vi "Add Sink.vi"(4 "Sink Name":string, 6 "Log Sink Reference":refnum<data-value>, 8 "error in (no error)":errorcluster, 11 "Application Log in":refnum<class "Application Log.lvclass">) -> (0 "error out":errorcluster, 3 "Application Log out":refnum<class "Application Log.lvclass">)   [LabVIEW 2016, in "Stream Log.lvlib" / "Application Log.lvclass"]
doc: "--\nCopyright © 2017 Composed SystemsI All rights reserved.\n\nAuthor: Jon McBee <jon.mcbee@composed.io>\n\nThis library is provided \"AS IS\" ,WITHOUT WARRANTIES OR\nCONDITIONS OF ANY KIND, either express or implied.\n\nComposed Systems -- composed.io\n\nStream 0.0.1.1\nJon McBee - Composed Systems\nCopyright (c) 2017, Composed Systems"
uses:
  <userlib>/Composed Systems/Stream/Log/Application Log/Application Log.lvclass
  <userlib>/Composed Systems/Stream/Log/Log Sink/Log Sink.lvclass
  <userlib>/Composed Systems/Stream/Log/Application Log/Application Log.lvclass/Application Log.ctl
  <userlib>/Composed Systems/Stream/Log/Sink Look Up Table/Sink Look Up Table.lvclass
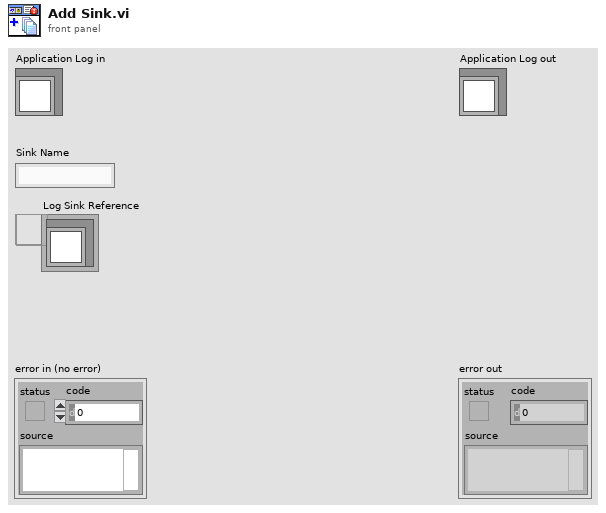
[diagram p1: front panel]
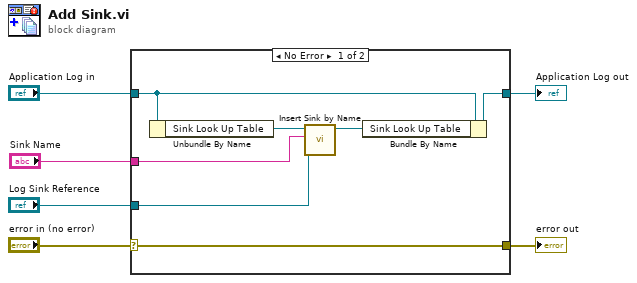
[diagram p0: block diagram]
diagram:
  n1 = case shown="No Error" "error in (no error)" {
    selector: "error in (no error)" -> [w13 w15]
    tunnel: [w13 w15] -> w5
    tunnel: [w11 w14] -> w3
    tunnel: "Application Log in" -> [w12 w14]
    tunnel: "Log Sink Reference" -> [w8 _]
    tunnel: "Sink Name" -> [w7 _]
    frame No Error {
      n2 = Unbundle By Name(w12) -> ("Sink Look Up Table"=w10:refnum<class "Sink Look Up Table.lvclass">)
      n3 = call <userlib>:"Insert Sink by Name.vi"("Log Sink"=w8, "Sink Name"=w7, "Sink Look Up Table in"=w10) -> ("Sink Look Up Table out"=w9:refnum<class "Sink Look Up Table.lvclass">)  [unwired: 6 in, 2 out]
      n4 = Bundle By Name(cluster=w12, "Sink Look Up Table"=w9) -> (w11:refnum<class "Application Log.lvclass">)
    }
    frame Error {
    }
  }
  "error out" <- w5
  "Application Log out" <- w3
